vi "Save settings to file.vi"(2 "DG measurement":T1={"Sampling frequencies (Hz)"=[10000000.0], "Requested PJVS frequencies (Hz)"=[1000.0], "Requested PJVS waveform amplitudes (V)"=[0.707], "Record lengths (multiples of PJVS periods)"=[10000.0], "Requested PJVS steps"=[20], "Switch position"=0.0, "Settle down after PJVS change (s)"=1.0, "Rs"=0, "Re"=0, "Algorithm"="TWM-PJVSSubS", "Calculate results"=FALSE, "Data folder"=path "", "TWM data directories"=[], "TWM data directories relative"=[], "DG measurement info files"=[], "Set PJVS frequencies (Hz)"=[1000.0], "Set PJVS reference voltages array of vector cluster"=[], "Set PJVS steps"=[1000]} {"Set PJVS frequencies (Hz)" format="%#_3p"; "Set PJVS reference voltages array of vector cluster"."PJVS reference voltages vector" format="%#_3p"; "Requested PJVS frequencies (Hz)" format="%#_3p"; "Record lengths (multiples of PJVS periods)" format="%#_3p"; "Sampling frequencies (Hz)" format="%#_3p"; "Requested PJVS waveform amplitudes (V)" format="%#_3p"}, 3 "AC sync source":T2, 4 "PJVS":T5={"PJVS type"=enum."AC-supraVOLTcontrol", "Status Refnum"=refnum, "AC-supraVOLTcontrol"={"IP address:port (0.0.0.0:0000)"="0.0.0.0:0000", "Timeouts"={"TCP Read & Write (ms)"=7000, "Sensors readout"=5000, "PJVS setup"=10000, "Nullmeter readout"=5000, "Multiplexer setup"=3000, "57XX setup"=15000, "Generator setup"=5000, "Synthesizer setup"=3000, "Sampler readout"=10000}, "Simulation mode"=FALSE, "Debug mode"=FALSE}, "NPL bias source"={"DataSocketCluster"={"Server Machine"="CZC105BD8M", "Client Machine"="localhost", "Data"="P2", "TimeStamp"=0.0, "Count"=1, "Target Process"="General Server"}}, "Manual PJVS"={"PJVS frequency (Hz)"=0.0, "Reference voltages (V)"=[], "File with PJVS voltages"=path ""}, "VTT PJVS"={"some VTT only property"=""}} {"NPL bias source"."DataSocketCluster"."TimeStamp" format="%.2f"}, 5 "SS measurement":T4={"Signal frequencies (Hz)"=[1000.0], "Signal amplitudes (V)"=[0.707], "Sampling frequencies (Hz)"=[10000000.0], "Record lengths (multiples of periods)"=[10000.0], "Calculate results"=FALSE, "Algorithm"="TWM-PJVSSubS", "TWM data directories"=[], "TWM data directories relative"=[], "Settle down after AC source change (s)"=1.0, "PJVS frequencies (Hz)"=[1000.0], "PJVS reference voltages array of vector cluster"=[{"PJVS reference voltages vector"=[]}], "Requested PJVS steps"=[20], "Measure CE"=FALSE, "Measure CE before"=FALSE, "Measure CE after"=FALSE, "Single point CE measurement"=FALSE, "original CE template path"=path "", "new CE template path before SS"=path "", "new CE template path before SS relative"=path "", "new CE template path after SS"=path "", "new CE template path after SS relative"=path "", "original CE fit path"=path "", "new CE fit path before SS"=path "", "new CE fit path before SS relative"=path "", "new CE fit path after SS"=path "", "new CE fit path after SS relative"=path "", "Measure digitizer gain"=FALSE, "Measure digitizer gain before"=FALSE, "Measure digitizer gain after"=FALSE, "Digitizer gain"=0.0, "Data folder"=path "", "FR fit path"=path "", "new FR fit path relative"=path "", "Rs"=0, "Re"=0, "SS measurement info files"=[]} {"PJVS reference voltages array of vector cluster"."PJVS reference voltages vector" format="%#_3p"; "PJVS frequencies (Hz)" format="%#_3p"; "Record lengths (multiples of periods)" format="%#_3p"; "Sampling frequencies (Hz)" format="%#_3p"; "Signal amplitudes (V)" format="%#_3p"; "Signal frequencies (Hz)" format="%#_3p"}, 6 "FR measurement":T9={"Measurement frequencies (Hz)"=[1000.0, 10000.0, 1000.0], "Sampling frequency (Hz)"=500000.0, "Signal amplitude (V)"=4.5, "AC-DC settle time (s)"=20.0, "Record length (multiples of period)"=[1000.0, 10000.0, 1000.0], "Measurement template file"=path "", "Row of START keyword"=0, "Row of STOP keyword"=0, "Calculate RMS from samples"=FALSE, "AC-DC warm up time (s)"=300.0, "Measurement template line"=[], "DC meter readings No."=10, "Algorithm"="TWM-WFFT", "Simultaneous measurement"=FALSE, "Recalculate-skip already calculated"=FALSE} {"Record length (multiples of period)" format="%#_3p"; "Sampling frequency (Hz)" format="%#_3p"; "Measurement frequencies (Hz)" format="%#_3p"}, 7 "CE measurement properties":T10={"Signal frequencies (Hz) T"=[1000.0], "Signal amplitudes (V) T"=[0.707], "Sampling frequencies (Hz) T"=[10000000.0], "Record lengths (multiples of periods) T"=[10000.0], "TWM data root directory"=path "", "TWM mreasurements directories"=[], "Calculate RMS from samples"=FALSE, "Algorithm to use"="TWM-WFFT", "Quantity to read"="TWM-WFFT", "Settle down after AC source change (s) T"=1.0, "Skip PJVS setup"=FALSE, "Measurement template file"=path "", "Row of START keyword T"=0, "Row of STOP keyword T"=0, "Measurement template line T"=[], "Switch position T"=[10000.0], "FR fit mat file T"=path "", "Recalculate-skip already calculated"=FALSE} {"Switch position T" format="%#_3p"; "Record lengths (multiples of periods) T" format="%#_3p"; "Sampling frequencies (Hz) T" format="%#_3p"; "Signal amplitudes (V) T" format="%#_3p"; "Signal frequencies (Hz) T" format="%#_3p"}, 8 "error in (no error)":errorcluster, 9 "DC meter":T11={"DC meter type"=enum."H/A/K 3458", "DC meter VISA"="", "NPLC"=10.0, "status ref"=refnum}, 10 "AC Source":T2, 11 "Common properties":T13={"Measurement status ref"=refnum, "TWM Status ref"=refnum, "Abort ref"=refnum, "Skip waiting ref"=refnum, "GNU Octave path"=path "C:/Program Files/GNU Octave/Octave-6.2.0/mingw64/bin", "TWM+QWTB path"=path "C:/Users/labina/Desktop/TWM-1.8.7.0-full/octprog", "lvlib path"=path "D:/martin/WAC/WACsw - github/control_software/Filter function meter/external libraries/GOLPI 0.7.3.1 source distribution LV 20.0 32 bit/lv_proc.dll", "TWM pipe"="\\\\.\\pipe\\TWM:server", "PJVS status ref"=refnum, "WAC path"=path ""}) -> (0 "error out":errorcluster)   [LabVIEW 2020]
uses:
  Type definitions/Common properties.ctl
  General AC source/Type definitions/AC Source.ctl
  General AC source/Type definitions/AC Source type.ctl
  General DC meter/Type definitions/DC meter.ctl
  General DC meter/Type definitions/DC meter type.ctl
  CE Measurement/Type definitions/CE measurement.ctl
  FR Measurement/Type definitions/FR measuement.ctl
  General PJVS driver/Type definitions/PJVS.ctl
  General PJVS driver/Type definitions/PJVS Type.ctl
  external libraries/acsvcontrol-driver/Public/Type Definitions/Timeouts.ctl
  external libraries/JV modified NPL Bias source/DataSocketCluster external.ctl
  SS Measurement/Type definitions/SS measurement.ctl
  DG Measurement/DG measurement.ctl
  <vilib>/Utility/xml.llb/Write to XML File(string).vi
  external libraries/acsvcontrol-driver/ACSVcontrol-driver.lvlib
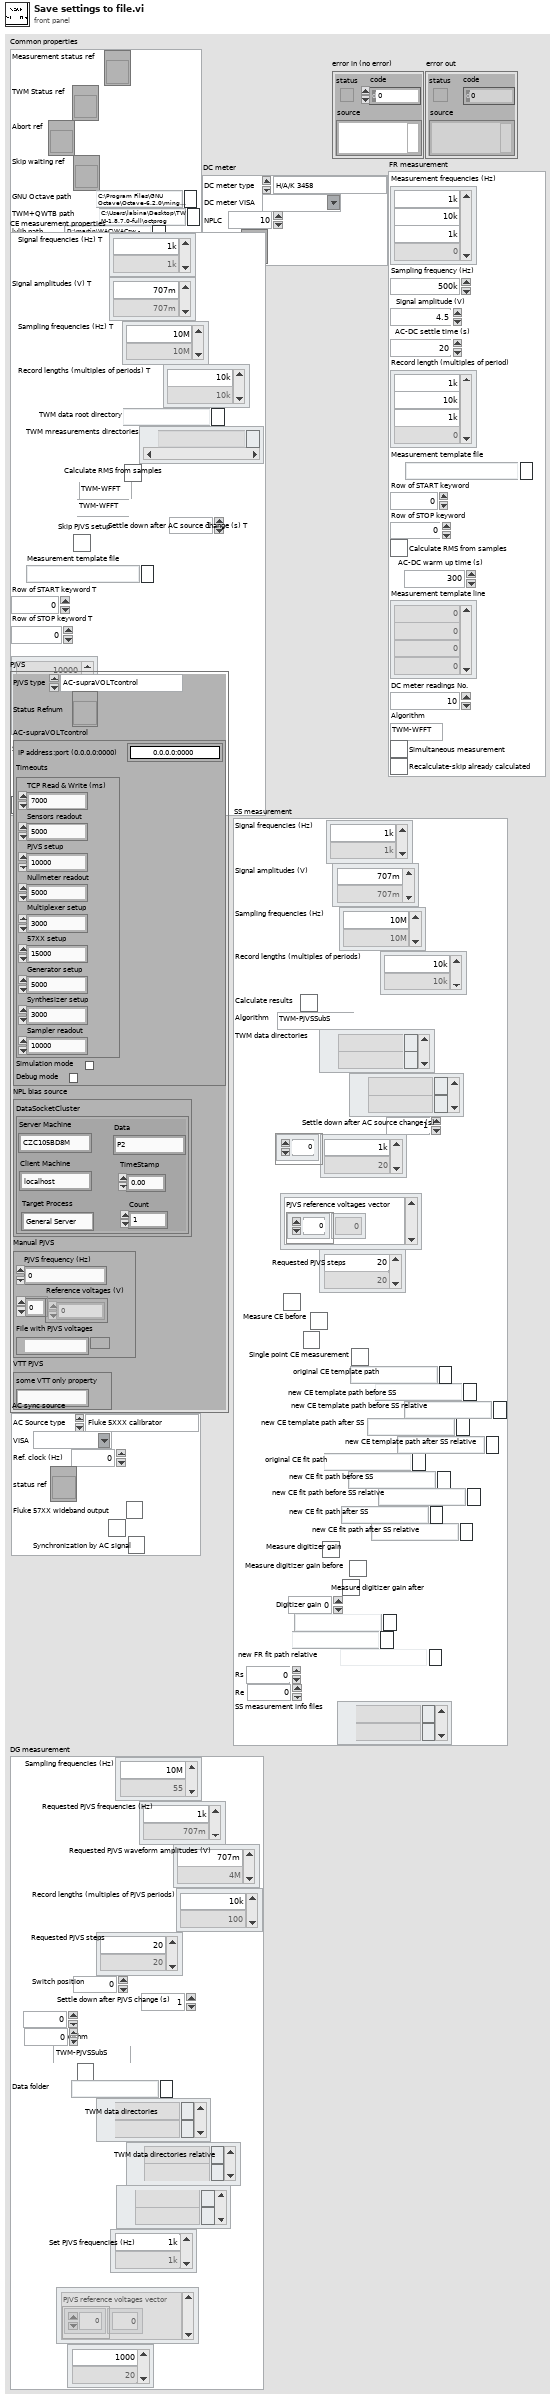
[diagram p1: front panel]
types:
  T1 = typedef "DG measurement.ctl" = cluster{"Sampling frequencies (Hz)":dbl[], "Requested PJVS frequencies (Hz)":dbl[], "Requested PJVS waveform amplitudes (V)":dbl[], "Record lengths (multiples of PJVS periods)":dbl[], "Requested PJVS steps":u32[], "Switch position":dbl, "Settle down after PJVS change (s)":dbl, "Rs":i32, "Re":i32, "Algorithm":string, "Calculate results":bool, "Data folder":path, "TWM data directories":path[], "TWM data directories relative":path[], "DG measurement info files":path[], "Set PJVS frequencies (Hz)":dbl[], "Set PJVS reference voltages array of vector cluster":cluster{"PJVS reference voltages vector":dbl[]}[], "Set PJVS steps":u32[]}
  T2 = typedef "AC Source.ctl" = cluster{"AC Source type":T3, "VISA":refnum<visa-resource-name>, "Ref. clock (Hz)":dbl, "status ref":refnum<vi>, "Fluke 57XX wideband output":bool, "Fluke 57XX ignore errors":bool, "Synchronization by AC signal":bool}
  T3 = typedef "AC Source type.ctl" = enum16{"Fluke 5XXX calibrator", "Tektronix AFG3000 series", "dummy", "Agilent 331xxA to 332xxA", "Agilent 335xxA to 336xxA"}
  T4 = typedef "SS measurement.ctl" = cluster{"Signal frequencies (Hz)":dbl[], "Signal amplitudes (V)":dbl[], "Sampling frequencies (Hz)":dbl[], "Record lengths (multiples of periods)":dbl[], "Calculate results":bool, "Algorithm":string, "TWM data directories":path[], "TWM data directories relative":path[], "Settle down after AC source change (s)":dbl, "PJVS frequencies (Hz)":dbl[], "PJVS reference voltages array of vector cluster":cluster{"PJVS reference voltages vector":dbl[]}[], "Requested PJVS steps":u32[], "Measure CE":bool, "Measure CE before":bool, "Measure CE after":bool, "Single point CE measurement":bool, "original CE template path":path, "new CE template path before SS":path, "new CE template path before SS relative":path, "new CE template path after SS":path, "new CE template path after SS relative":path, "original CE fit path":path, "new CE fit path before SS":path, "new CE fit path before SS relative":path, "new CE fit path after SS":path, "new CE fit path after SS relative":path, "Measure digitizer gain":bool, "Measure digitizer gain before":bool, "Measure digitizer gain after":bool, "Digitizer gain":dbl, "Data folder":path, "FR fit path":path, "new FR fit path relative":path, "Rs":i32, "Re":i32, "SS measurement info files":path[]}
  T5 = typedef "PJVS.ctl" = cluster{"PJVS type":T6, "Status Refnum":refnum<vi>, "AC-supraVOLTcontrol":cluster{"IP address:port (0.0.0.0:0000)":string, "Timeouts":T7, "Simulation mode":bool, "Debug mode":bool}, "NPL bias source":cluster{"DataSocketCluster":T8}, "Manual PJVS":cluster{"PJVS frequency (Hz)":dbl, "Reference voltages (V)":dbl[], "File with PJVS voltages":path}, "VTT PJVS":cluster{"some VTT only property":string}}
  T6 = typedef "PJVS Type.ctl" = enum16{"AC-supraVOLTcontrol", "JV modified NPL bias control", "Manual PJVS", "VTT PJVS"}
  T7 = typedef "ACSVcontrol-driver.lvlib/Timeouts.ctl" = cluster{"TCP Read & Write (ms)":i32, "Sensors readout":i32, "PJVS setup":i32, "Nullmeter readout":i32, "Multiplexer setup":i32, "57XX setup":i32, "Generator setup":i32, "Synthesizer setup":i32, "Sampler readout":i32}
  T8 = typedef "DataSocketCluster external.ctl" = cluster{"Server Machine":string, "Client Machine":string, "Data":string, "TimeStamp":dbl, "Count":i32, "Target Process":string}
  T9 = typedef "FR measuement.ctl" = cluster{"Measurement frequencies (Hz)":dbl[], "Sampling frequency (Hz)":dbl, "Signal amplitude (V)":dbl, "AC-DC settle time (s)":dbl, "Record length (multiples of period)":dbl[], "Measurement template file":path, "Row of START keyword":i32, "Row of STOP keyword":i32, "Calculate RMS from samples":bool, "AC-DC warm up time (s)":dbl, "Measurement template line":i32[], "DC meter readings No.":i32, "Algorithm":string, "Simultaneous measurement":bool, "Recalculate-skip already calculated":bool}
  T10 = typedef "CE measurement.ctl" = cluster{"Signal frequencies (Hz) T":dbl[], "Signal amplitudes (V) T":dbl[], "Sampling frequencies (Hz) T":dbl[], "Record lengths (multiples of periods) T":dbl[], "TWM data root directory":path, "TWM mreasurements directories":path[], "Calculate RMS from samples":bool, "Algorithm to use":string, "Quantity to read":string, "Settle down after AC source change (s) T":dbl, "Skip PJVS setup":bool, "Measurement template file":path, "Row of START keyword T":i32, "Row of STOP keyword T":i32, "Measurement template line T":i32[], "Switch position T":dbl[], "FR fit mat file T":path, "Recalculate-skip already calculated":bool}
  T11 = typedef "DC meter.ctl" = cluster{"DC meter type":T12, "DC meter VISA":refnum<visa-resource-name>, "NPLC":dbl, "status ref":refnum<vi>}
  T12 = typedef "DC meter type.ctl" = enum16{"H/A/K 3458", "Fluke 8508A", "dummy", "Keithley 2182"}
  T13 = typedef "Common properties.ctl" = cluster{"Measurement status ref":refnum<vi>, "TWM Status ref":refnum<vi>, "Abort ref":refnum<vi>, "Skip waiting ref":refnum<vi>, "GNU Octave path":path, "TWM+QWTB path":path, "lvlib path":path, "TWM pipe":string, "PJVS status ref":refnum<vi>, "WAC path":path}
  T14 = typedef "Type definitions to be saved.ctl" = cluster{"Common properties":T13, "AC Source":T2, "DC meter":T11, "CE measurement":T10, "FR measurement":T9, "FR template":T15, "CE template":T16, "PJVS":T5, "SS measurement":T4, "AC sync source":T2, "DG measurement":T1}
  T15 = typedef "FR template.ctl" = cluster{"Keywords column":i32, "Sig. freq. column":i32, "Rec. len. column":i32, "Meas. points. row min to read":i32, "Meas. points. row max to read":i32, "Properties column":i32, "Properties row start":i32, "Properties row end":i32, "Keyword START regexp":string, "Keyword STOP regexp":string, "HW data column":i32, "HW data row start":i32, "HW data row end":i32, "TIme and date column start":i32, "Digitizer value column start ":i32, "DC mean column start ":i32, "DC readings column start":i32}
  T16 = typedef "CE template.ctl" = cluster{"Keywords column":i32, "Sig. freq. column":i32, "Rec. len. column":i32, "Switch pos column":i32, "Meas. points. row min to read":i32, "Meas. points. row max to read":i32, "Properties column":i32, "Properties row start":i32, "Properties row end":i32, "Keyword START regexp":string, "Keyword STOP regexp":string, "HW data column":i32, "HW data row start":i32, "HW data row end":i32, "TIme and date column start":i32, "Digitizer value column start ":i32}
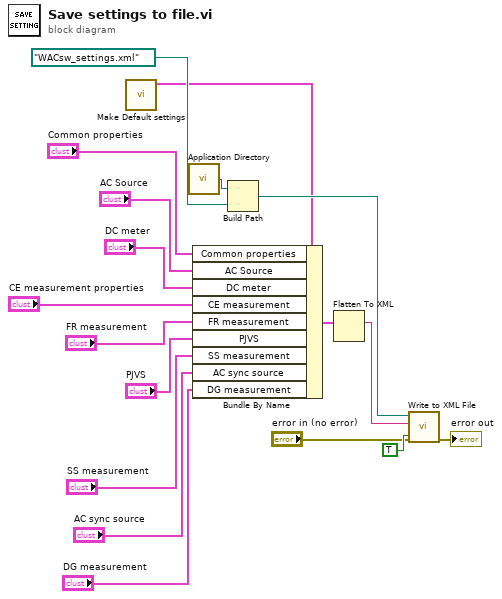
[diagram p0: block diagram]
diagram:
  n1 = call "Make Default settings.vi"() -> ("TD to be saved"=w11:T14)  [unwired: 11 in]
  n2 = call <vilib>:"Application Directory.vi"() -> ("Application Directory"=w16:path)
  n3 = Bundle By Name(cluster=w11, "Common properties"="Common properties", "AC Source"="AC Source", "DC meter"="DC meter", "CE measurement"="CE measurement properties", "FR measurement"="FR measurement", "PJVS"="PJVS", "SS measurement"="SS measurement", "AC sync source"="AC sync source", "DG measurement"="DG measurement") -> (w6:T14)
  n4 = Build Path(base path=w16, name or relative path=path "WACsw_settings.xml") -> (appended path=w14:path)
  n5 = Flatten To XML(6:w6) -> (2:w18:string)
  n6 = call-poly <vilib>:"Write to XML File.vi"("Standalone? (T)"=TRUE, "error in (no error)"="error in (no error)", "XML Input"=w18, "XML File Path"=w14) -> ("error out"=→"error out":errorcluster)  [unwired: 5 in, 2 out]
